vi "B侧下降（Trans).vi"(8 "error in (no error)":errorcluster caption="错误输入（无错误）", 11 "Data In":T1) -> (0 "error out":errorcluster caption="错误输出", 3 "Data Out":T1)   [LabVIEW 2013]
uses:
  Control/Data.ctl
  Control/YV.ctl
  Control/SW.ctl
  Control/State.ctl
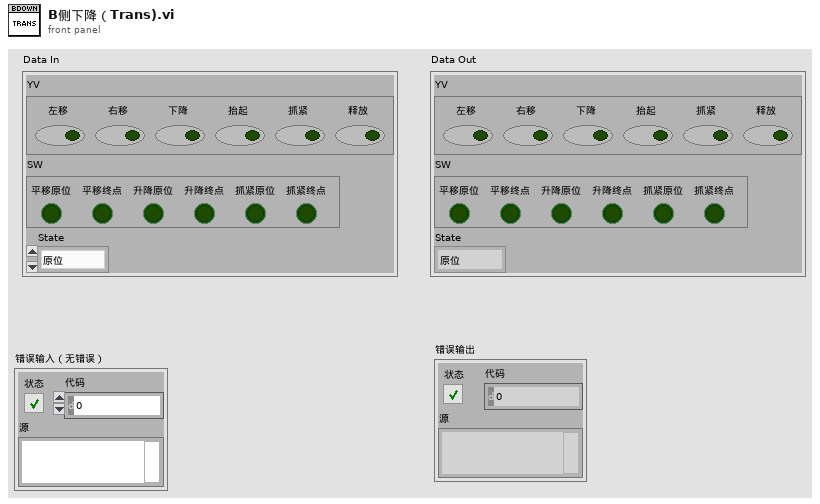
[diagram p1: front panel]
types:
  T1 = typedef "Data.ctl" = cluster{"YV":T2, "SW":T3, "State":T4}
  T2 = typedef "YV.ctl" = cluster{"左移":bool, "右移":bool, "下降":bool, "抬起":bool, "抓紧":bool, "释放":bool}
  T3 = typedef "SW.ctl" = cluster{"平移原位":bool, "平移终点":bool, "升降原位":bool, "升降终点":bool, "抓紧原位":bool, "抓紧终点":bool}
  T4 = typedef "State.ctl" = enum16{"原位", "A侧下降", "夹紧工件", "A侧抬起", "右移", "B侧下降", "释放工件", "B侧抬起", "左移"}
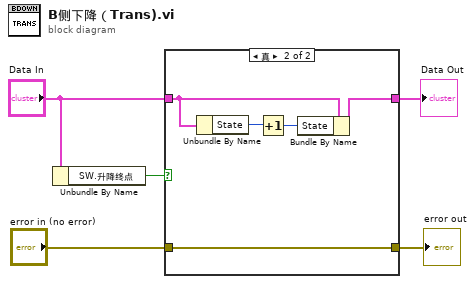
[diagram p0: block diagram]
diagram:
  n1 = Unbundle By Name("Data In") -> ("SW.升降终点"=w2:bool)
  n2 = case shown="真" w2 {
    tunnel: "error in (no error)" -> [w7 w12]
    tunnel: [w7 w12] -> w4
    tunnel: [w6 w10] -> w1
    tunnel: "Data In" -> [w6 w9]
    frame False {
    }
    frame True {
      n3 = Unbundle By Name(w9) -> ("State"=w8:T4)
      n4 = Increment(x=w8) -> (x+1=w11:T4)
      n5 = Bundle By Name(cluster=w9, "State"=w11) -> (w10:T1)
    }
  }
  "Data Out" <- w1
  "error out" <- w4
